vi "Init_Lawicel.vi"(1 "baud":u16(ring)=20 items=["1M"=20, "500K"=28, "250K"=284, "125K"=796, "100K"=17199, "50K"=18223, "20K"=21295, "10K"=26415, "5K"=32639], 2 "Seria- Port":refnum<visa-resource-name>="COM5") -> (3 "error out 4":errorcluster, 4 "Status":bool, 5 "read ver":string, 6 "VISA res_out":refnum<visa-resource-name>)   [LabVIEW 2010]
uses:
  <vilib>/Instr/_visa.llb/VISA Configure Serial Port (Instr).vi
panel:
  out "error out":errorcluster
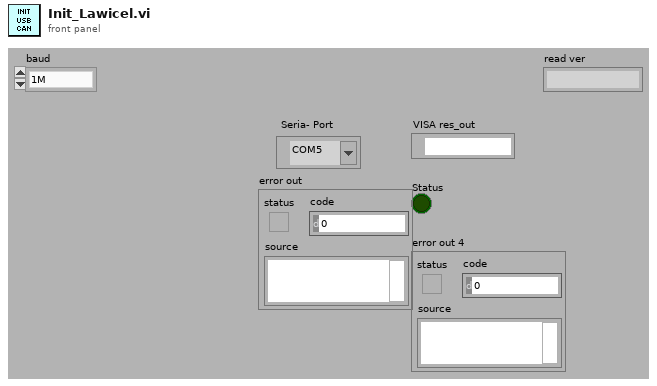
[diagram p1: front panel]
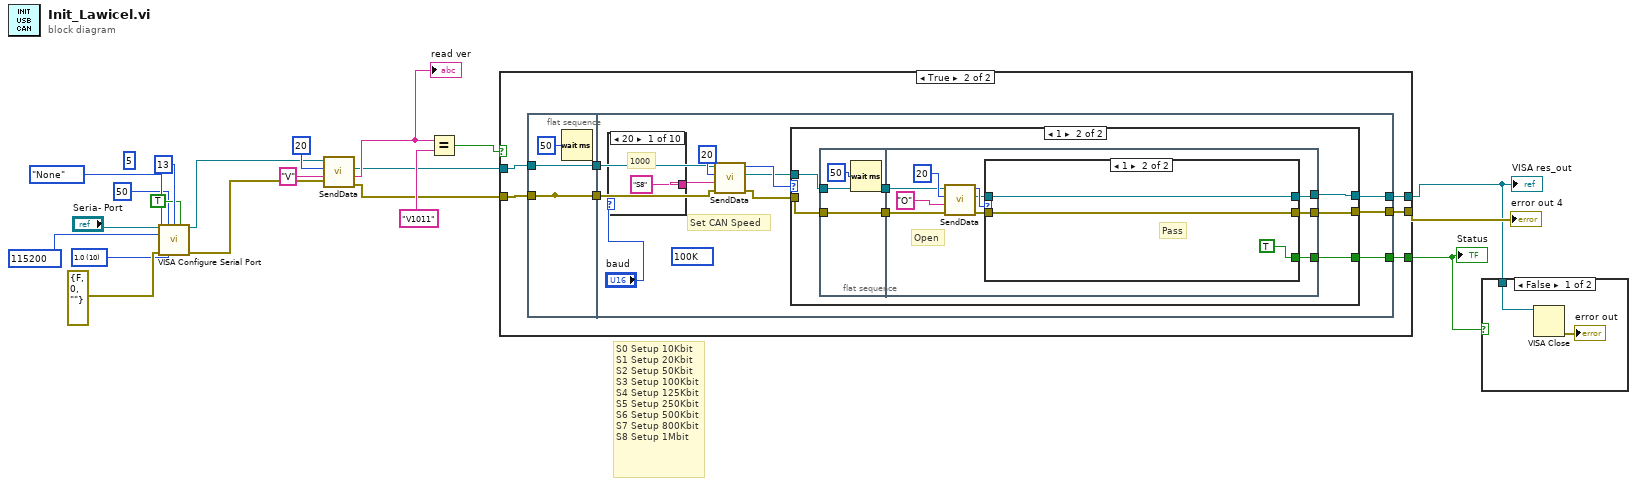
[diagram p0: block diagram]
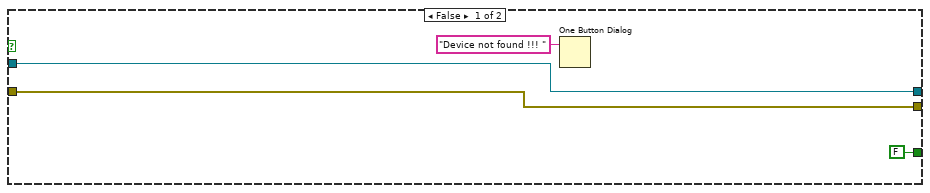
[diagram p3: hidden frame]
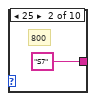
[diagram p4: hidden frame]
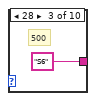
[diagram p5: hidden frame]
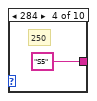
[diagram p6: hidden frame]
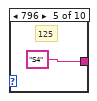
[diagram p7: hidden frame]
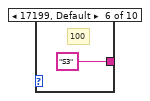
[diagram p8: hidden frame]
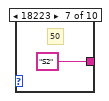
[diagram p9: hidden frame]
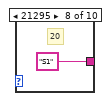
[diagram p10: hidden frame]
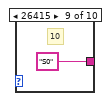
[diagram p11: hidden frame]
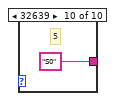
[diagram p12: hidden frame]
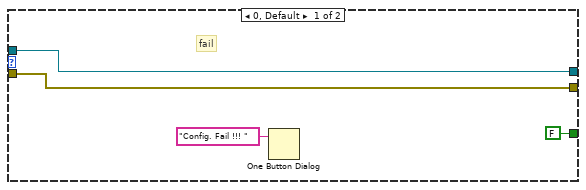
[diagram p13: hidden frame]
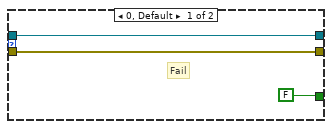
[diagram p14: hidden frame]
diagram:
  w11 = u32 115200 items=["4800"=4800, "9600"=9600, "19200"=19200, "38400"=38400, "57600"=57600, "115200"=115200] ("Baud rate")
  w12 = u16 10 items=["1.0"=10, "1.5"=15, "2.0"=20] ("stop bits")
  (unwired) u32 5 ("timeout (10sec)")
  # "S0 Setup 10Kbit\nS1 Setup 20Kbit\nS2 Setup 50Kbit\nS3 Setup 100Kbit\nS4 Setup 125Kbit\nS5 Setup 250Kbit\nS6 Setup 500Kbit\nS7 Setup 800Kbit\nS8 Setup 1Mbit"
  n1 = call-poly "VISA Configure Serial Port"("VISA resource name"="Seria- Port", "timeout (10sec)"=u32 50, "termination char\n(0xA = '\\n' = LF)"=u8 13 ("termination char\n(0xA = '\\n' = LF)"), "Enable Termination\nChar (T)"=TRUE ("Enable Termination\nChar (T)"), "baud rate (9600)"=w11, "parity (0:none)"=enum16{"None", "Odd", "Even", "Mark", "Space"}."None", "error in (no error)"=errorcluster {"status"=FALSE, "code"=0, "source"=""} ("error in"), "stop bits (10: 1 bit)"=w12) -> ("VISA resource name out"=w13:refnum<visa-resource-name>, "error out"=w14:errorcluster)  [unwired: 6 in]
  n2 = call "SendData.vi"("error out 2"=w14, "String"="V", "byte count"=u32 20, "VISA resource name out 2"=w13) -> ("error out"=w6:errorcluster, "read buffer"=w19:string, "VISA resource name out"=w5:refnum<visa-resource-name>)  [unwired: 1 out]
  "read ver" <- w19
  n3 = Equal?(x=w19, y="V1011") -> (x = y?=w7:bool)
  n4 = case shown="True" w7 {
    tunnel: w6 -> [w22 w29]
    tunnel: w5 -> [w23 w28]
    tunnel: [w23 w27] -> w2
    tunnel: [w22 w26] -> w4
    tunnel: [FALSE ("Status") w25] -> w3
    frame False {
      n5 = One Button Dialog(message="Device not found !!! ") -> ()  [unwired: 1 in, 1 out]
    }
    frame True {
      n6 = flat-sequence {
        tunnel: [w32] -> _
        tunnel: w28 -> [w34]
        tunnel: [w34] -> w31
        tunnel: [w32] -> w30
        tunnel: w29 -> [w32]
        tunnel: w31 -> [w44]
        tunnel: w30 -> [w43]
        tunnel: [w38] -> w27
        tunnel: [w39] -> w26
        tunnel: [w37] -> w25
        frame #0 {
          n7 = Wait (ms)(milliseconds to wait=u32 50) -> ()  [unwired: 1 out]
        }
        frame #1 {
          (unwired) u16 17199 items=["1M"=20, "500K"=28, "250K"=284, "125K"=796, "100K"=17199, "50K"=18223, "20K"=21295, "10K"=26415, "5K"=32639] ("baud 2")
          # "Set CAN Speed"
          n8 = case shown="20" "baud" {
            tunnel: ["S8" "S7" "S6" "S5" "S4" "S3" "S2" "S1" "S0" "S0"] -> w36
            frame 20 {
              # "1000"
            }
            frame 25 {
              # "800"
            }
            frame 28 {
              # "500"
            }
            frame 284 {
              # "250"
            }
            frame 796 {
              # "125"
            }
            frame 17199, Default {
              # "100"
            }
            frame 18223 {
              # "50"
            }
            frame 21295 {
              # "20"
            }
            frame 26415 {
              # "10"
            }
            frame 32639 {
              # "5"
            }
          }
          n9 = call "SendData.vi"("error out 2"=w43, "String"=w36, "byte count"=u32 20, "VISA resource name out 2"=w44) -> ("error out"=w40:errorcluster, "VISA resource name out"=w41:refnum<visa-resource-name>, "status_1_OK"=w42:i32)  [unwired: 1 out]
          n10 = case shown="1" w42 {
            tunnel: w41 -> [w58 w65]
            tunnel: w40 -> [w57 w66]
            tunnel: [w58 w62] -> w38
            tunnel: [w57 w61] -> w39
            tunnel: [FALSE ("Status") w60] -> w37
            frame 0, Default {
              # "fail"
              n11 = One Button Dialog(message="Config. Fail !!! ") -> ()  [unwired: 1 in, 1 out]
            }
            frame 1 {
              n12 = flat-sequence {
                tunnel: w65 -> [w68]
                tunnel: w66 -> [w69]
                tunnel: [w69] -> w64
                tunnel: [w68] -> w63
                tunnel: w64 -> [w78]
                tunnel: w63 -> [w76]
                tunnel: [w72] -> w62
                tunnel: [w71] -> w61
                tunnel: [w70] -> w60
                frame #0 {
                  n13 = Wait (ms)(milliseconds to wait=u32 50) -> ()  [unwired: 1 out]
                }
                frame #1 {
                  # "Open"
                  n14 = call "SendData.vi"("error out 2"=w78, "String"="O", "byte count"=u32 20, "VISA resource name out 2"=w76) -> ("error out"=w73:errorcluster, "VISA resource name out"=w74:refnum<visa-resource-name>, "status_1_OK"=w75:i32)  [unwired: 1 out]
                  n15 = case shown="1" w75 {
                    tunnel: w74 -> [w82 w85]
                    tunnel: [w82 w85] -> w72
                    tunnel: w73 -> [w81 w84]
                    tunnel: [w81 w84] -> w71
                    tunnel: [FALSE ("Status") TRUE ("Status")] -> w70
                    frame 0, Default {
                      # "Fail"
                    }
                    frame 1 {
                      # "Pass"
                    }
                  }
                }
              }
            }
          }
        }
      }
    }
  }
  "VISA res_out" <- w2
  "error out 4" <- w4
  "Status" <- w3
  n16 = case shown="False" w3 {
    tunnel: w2 -> [w87 _]
    frame False {
      n17 = VISA Close(VISA resource name=w87) -> (error out=→"error out":errorcluster)  [unwired: 1 in]
    }
    frame True {
    }
  }
